vi "TCP Msg Server.vi"() -> ()   [LabVIEW 2020]
uses:
  <vilib>/IlluminatedG/lv-stream-tcp/TCP Server/TCP Server.lvclass
  <vilib>/IlluminatedG/lv-stream/Endpoint/Endpoint.lvclass
  Manager/Manager.lvclass
  C:/Program Files (x86)/National Instruments/LabVIEW 2020/vi.lib/IlluminatedG/lv-stream/Endpoint/Endpoint.lvclass
  C:/Program Files (x86)/National Instruments/LabVIEW 2020/vi.lib/IlluminatedG/lv-stream-tcp/TCP Server/TCP Server.lvclass
  b5c60ef6-5327-461d-804d-ec976e821dd3.vi
  f62ccf13-e430-49b0-9820-5d38b530824a.vi
panel:
  out "error out":errorcluster
  in  "Slide":dbl(slide) scale=0.0..10.0
  in  "Stop":bool
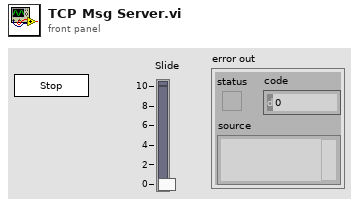
[diagram p1: front panel]
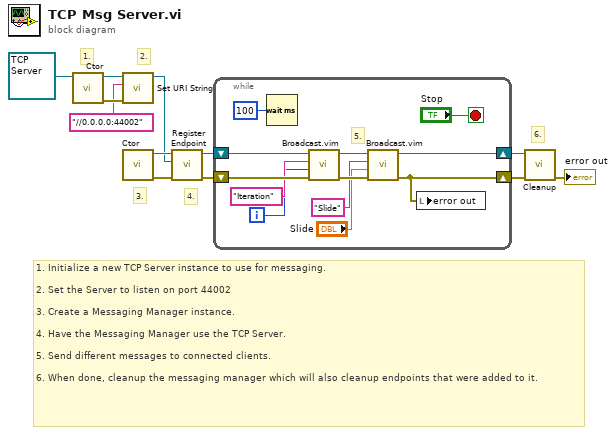
[diagram p0: block diagram]
diagram:
  # "6."
  # "1. Initialize a new TCP Server instance to use for messaging.\n\n2. Set the Server to listen on port 44002\n\n3. Create a Messaging Manager instance.\n\n4. Have the Messaging Manager use the TCP Server.\n\n5. Send different messages to connected clients.\n\n6. When done, cleanup the messaging manager which will also cleanup endpoints that were added to it."
  # "4."
  # "3."
  # "2."
  # "1."
  n1 = call-dynamic "Ctor.vi"("TCP Server in"=refnum<class "TCP Server.lvclass"> refnum) -> ("error out"=w9:errorcluster, "TCP Server out"=w10:refnum<class "TCP Server.lvclass">)  [unwired: 9 in]
  n2 = call <vilib>:"Set URI String.vi"("error in (no error)"=w9, "URI String"="//0.0.0.0:44002", "Endpoint in"=w10) -> ("Endpoint out"=w1:refnum<class "TCP Server.lvclass">)  [unwired: 7 in, 1 out]
  n3 = call "Ctor.vi"() -> ("error out"=w4:errorcluster, "Manager out"=w7:refnum<class "Manager.lvclass">)  [unwired: 10 in]
  n4 = call "Register Endpoint.vi"("error in (no error)"=w4, "Stream:Endpoint"=w1, "Manager in"=w7) -> ("error out"=w12:errorcluster, "Manager out"=w6:refnum<class "Manager.lvclass">)  [unwired: 7 in]
  n5 = while {
    shift-right: [w15] -> w5
    shift-left: w6 -> [w23]
    shift-right: [w13] -> w3
    shift-left: w12 -> [w24]
    i -> [w21]
    stop <- "Stop" stop-if-true
    # "5."
    n6 = Wait (ms)(milliseconds to wait=u32 100) -> ()  [unwired: 1 out]
    n7 = call "Broadcast.vim"("error in (no error)"=w24, "Data (With ID String)"=w21, "Message (Or ID String)"="Iteration", "Manager in"=w23) -> ("error out"=w18:errorcluster, "Manager out"=w19:refnum<class "Manager.lvclass">)  [unwired: 6 in]
    n8 = call "Broadcast.vim"("error in (no error)"=w18, "Data (With ID String)"="Slide", "Message (Or ID String)"="Slide", "Manager in"=w19) -> ("error out"=w13:errorcluster, "Manager out"=w15:refnum<class "Manager.lvclass">)  [unwired: 6 in]
    n9 = local write "error out"(w13) -> ()
  }
  n10 = call "Cleanup.vi"("error in (no error)"=w3, "Manager in"=w5) -> ("error out"=→"error out":errorcluster)  [unwired: 9 in]
